vi "DecodeYPRUpdate.vi"(11 "Buffer":string) -> (3 "MessageReceived":bool)   [LabVIEW 2014, in "Nav6.lvlib"]
uses:
  Nav6.lvlib
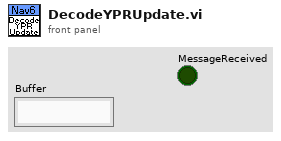
[diagram p1: front panel]
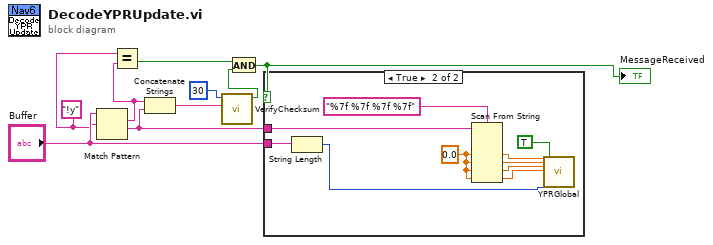
[diagram p0: block diagram]
diagram:
  w5 = "!y" ("string")
  n1 = Match Pattern(string="Buffer", regular expression=w5) -> (match substring=w4:string, after substring=w9:string)  [unwired: 1 in, 2 out]
  n2 = Equal?(x=w5, y=w4) -> (x = y?=w1:bool)
  n3 = Concatenate Strings(w4, w9) -> (w7:string)
  n4 = call "VerifyChecksum.vi"("String"=w7, "ChecksumIndex"=30) -> ("ChecksumVerified"=w3:bool)  [unwired: 9 in]
  n5 = And(x=w1, y=w3) -> (x .and. y?=w2:bool)
  "MessageReceived" <- w2
  n6 = case shown="True" w2 {
    tunnel: w9 -> [_ w19]
    tunnel: "Buffer" -> [_ w11]
    frame False {
    }
    frame True {
      w17 = 0.0 ("default value 1")
      n7 = String Length(string=w11) -> (length=w10:i32)
      n8 = Scan From String(format string="%7f %7f %7f %7f", input string=w19, default 1=w17, default 2=w17, default 3=w17, default 4=w17) -> (output 1=w16:dbl, output 2=w15:dbl, output 3=w14:dbl, output 4=w13:dbl)  [unwired: 2 in, 3 out]
      n9 = call "YPRGlobal.vi"("Yaw"=w16, "Pitch"=w15, "Roll"=w14, "Compass Heading"=w13, "Byte Count"=w10, "Update"=TRUE) -> ()  [unwired: 15 in, 7 out]
    }
  }
